vi "Multiply CFX4.21 by BPSK Symbol.vi"(9 "BPSK symbol":T2={"BPSK constellation"=TRUE, "not in list"=TRUE}, 10 "subcarrier in":T1) -> (2 "subcarrier out":T1)   [LabVIEW 2020]
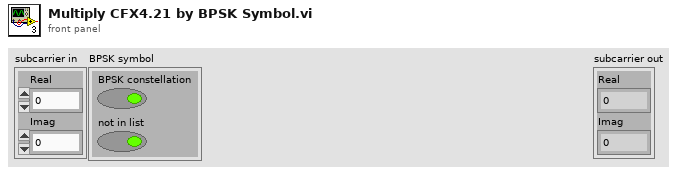
[diagram p1: front panel]
types:
  T1 = cluster{"Real":fxp<+/-,25,4>, "Imag":fxp<+/-,25,4>}
  T2 = cluster{"BPSK constellation":bool, "not in list":bool}
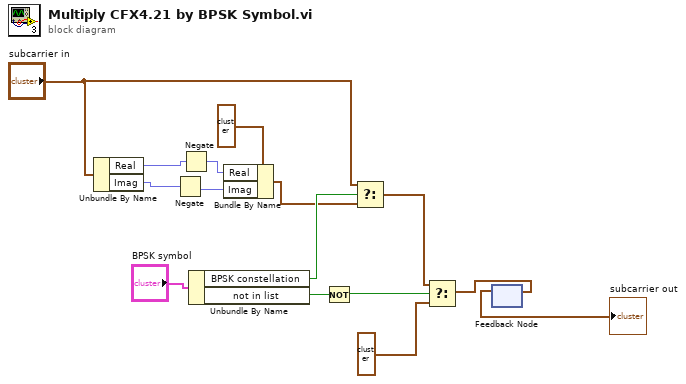
[diagram p0: block diagram]
diagram:
  n1 = Unbundle By Name("subcarrier in") -> ("Real"=w7:fxp<+/-,25,4>, "Imag"=w6:fxp<+/-,25,4>)
  n2 = Negate(x=w6) -> (-x=w4:fxp<+/-,25,4>)
  n3 = Negate(x=w7) -> (-x=w5:fxp<+/-,25,4>)
  n4 = Unbundle By Name("BPSK symbol") -> ("BPSK constellation"=w14:bool, "not in list"=w13:bool)
  n5 = Bundle By Name(cluster=T1 {"Real"=0.0, "Imag"=0.0} ("subcarrier in"), "Real"=w5, "Imag"=w4) -> (w2:T1)
  n6 = Not(x=w13) -> (.not. x?=w12:bool)
  n7 = Select(t="subcarrier in", s=w14, f=w2) -> (s? t:f=w11:T1)
  n8 = Select(t=w11, s=w12, f=T1 {"Real"=0.0, "Imag"=0.0} ("subcarrier in")) -> (s? t:f=w10:T1)
  n9 = feedback-in #1(w10) -> ()
  n10 = feedback #1() -> (→"subcarrier out":T1)  [unwired: 1 in]
